vi "Periodic 1-Exp Distributed Random Variable.vi"(6 "seed":i32=-1, 8 "Error In":errorcluster, 9 "T":dbl, 10 "tau":dbl, 11 "# Elements":i32) -> (0 "Error Out":errorcluster, 3 "t Array":dbl[](array[numeric]))   [LabVIEW 2021, in "Math.lvlib"]
uses:
  Math.lvlib
  <vilib>/Utility/error.llb/Error Cluster From Error Code.vi
  <vilib>/gmath/statdist.llb/Uniform Random.vi
  <vilib>/ErrorRing/Error Ring.xnode
  <vilib>/gmath/NI_Gmath.lvlib
  Error/Error.lvlib
  Comparison/Comparison.lvlib
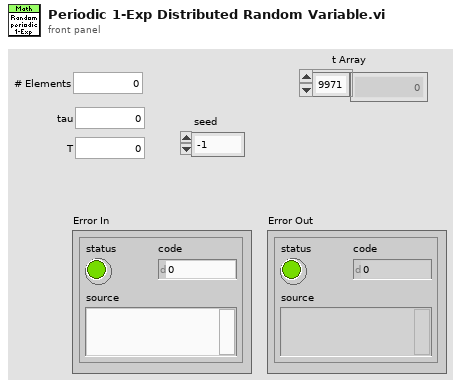
[diagram p1: front panel]
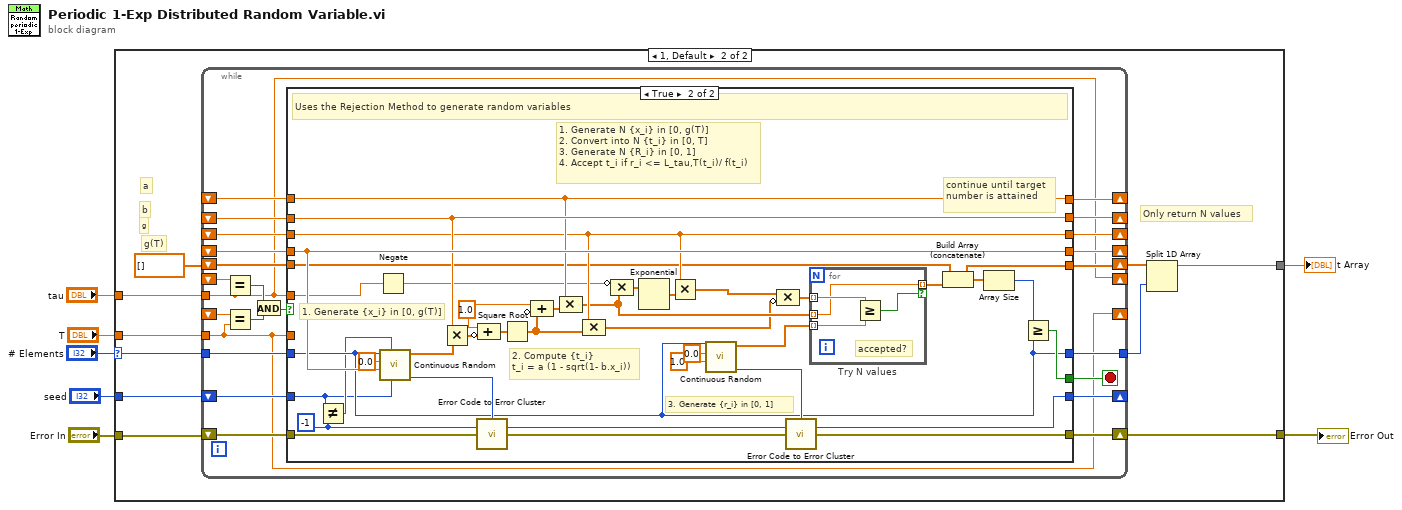
[diagram p0: block diagram]
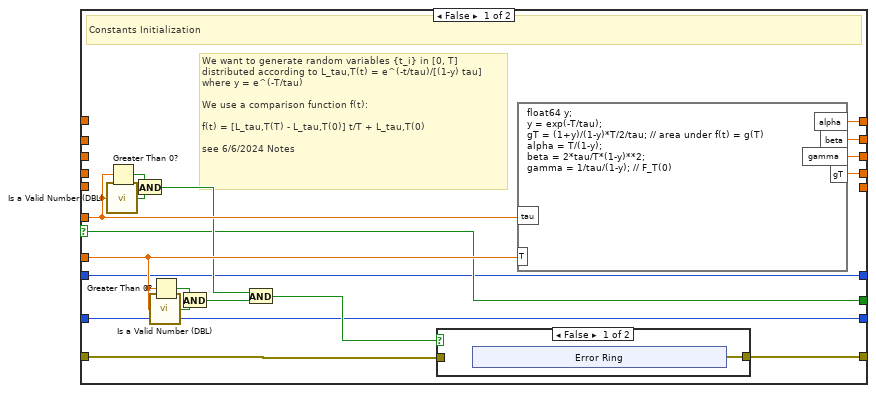
[diagram p3: hidden frame]
diagram:
  n1 = case shown="1, Default" "# Elements" {
    selector: "# Elements" -> [_ w16]
    tunnel: "tau" -> [_ w18]
    tunnel: "T" -> [_ w17]
    tunnel: "seed" -> [_ w15]
    tunnel: "Error In" -> [w8 w14]
    tunnel: [w8 w13] -> w2
    tunnel: [_ w10] -> w1
    frame 0 {
    }
    frame 1, Default {
      # "Only return N values"
      # "a"
      # "g"
      # "b"
      # "g(T)"
      n2 = while {
        tunnel: w18 -> [w19]
        shift-right: [w19] -> _
        shift-left: _ -> [w42]
        tunnel: w17 -> [w20]
        shift-right: [w20] -> _
        shift-left: _ -> [w41]
        shift-right: [w37] -> _
        shift-left: _ -> [w36]
        tunnel: w16 -> [w35]
        shift-right: [w34] -> _
        shift-left: _ -> [w32]
        shift-right: [w33] -> _
        shift-left: _ -> [w31]
        shift-right: [w28] -> w13
        shift-left: w14 -> [w29]
        shift-right: [w27] -> _
        shift-left: _ -> [w26]
        shift-right: [w23] -> w12
        shift-left: dbl[] [] -> [w24]
        tunnel: [w22] -> w11
        shift-right: [w21] -> _
        shift-left: w15 -> [w30]
        stop <- w25 stop-if-true
        n3 = Equal?(x=w42, y=w19) -> (x = y?=w39:bool)
        n4 = Equal?(x=w41, y=w20) -> (x = y?=w40:bool)
        n5 = And(x=w39, y=w40) -> (x .and. y?=w38:bool)
        n6 = case shown="True" w38 {
          selector: w38 -> [w45 _]
          tunnel: w19 -> [w57 w89]
          tunnel: w20 -> [w56 _]
          tunnel: [w60 w101] -> w37
          tunnel: w36 -> [_ w101]
          tunnel: w35 -> [w44 w73]
          tunnel: [w59 w99] -> w34
          tunnel: [w58 w90] -> w33
          tunnel: w32 -> [_ w99]
          tunnel: w31 -> [_ w90]
          tunnel: w30 -> [w43 w71]
          tunnel: w29 -> [w48 w69]
          tunnel: [w47 w67] -> w28
          tunnel: [w46 w92] -> w27
          tunnel: w26 -> [_ w92]
          tunnel: [w45 w84] -> w25
          tunnel: w24 -> [_ w86]
          tunnel: [_ w83] -> w23
          tunnel: [w44 w73] -> w22
          tunnel: [w43 w70] -> w21
          frame False {
            # "We want to generate random variables {t_i} in [0, T]\ndistributed according to L_tau,T(t) = e^(-t/tau)/[(1-y) tau]\nwhere y = e^(-T/tau)\n\nWe use a comparison function f(t):\n\nf(t) = [L_tau,T(T) - L_tau,T(0)] t/T + L_tau,T(0)\n\nsee 6/6/2024 Notes"
            # "Constants Initialization"
            n7 = call "Is a Valid Number (DBL).vi"("Number"=w57) -> ("Valid Number?"=w54:bool)  [unwired: 8 in]
            n8 = Greater Than 0?(x=w57) -> (x > 0?=w55:bool)
            n9 = And(x=w55, y=w54) -> (x .and. y?=w50:bool)
            n10 = call "Is a Valid Number (DBL).vi"("Number"=w56) -> ("Valid Number?"=w52:bool)  [unwired: 8 in]
            n11 = Greater Than 0?(x=w56) -> (x > 0?=w53:bool)
            n12 = And(x=w53, y=w52) -> (x .and. y?=w51:bool)
            n13 = And(x=w50, y=w51) -> (x .and. y?=w49:bool)
            n14 = case shown="False" w49 {
              tunnel: w48 -> [_ w66]
              tunnel: [w61 w66] -> w47
              frame False {
                n15 = xnode "Error Ring"() -> ("error out"=w61:errorcluster)
              }
              frame True {
              }
            }
            n16 = formula code="float64 y;\ny = exp(-T/tau);\ngT = (1+y)/(1-y)*T/2/tau; // area under f(t) = g(T)\nalpha = T/(1-y);\nbeta = 2*tau/T*(1-y)**2;\ngamma = 1/tau/(1-y); // F_T(0)"("tau"=w57, "T"=w56) -> ("gT"=w60:dbl, "beta"=w59:dbl, "gamma"=w58:dbl, "alpha"=w46:dbl)
          }
          frame True {
            w70 = -1 ("x")
            w94 = 1.0 ("xmin")
            # "3. Generate {r_i} in [0, 1]"
            # "2. Compute {t_i}\nt_i = a (1 - sqrt(1- b.x_i))"
            # "1. Generate {x_i} in [0, g(T)]"
            # "1. Generate N {x_i} in [0, g(T)]\n2. Convert into N {t_i} in [0, T]\n3. Generate N {R_i} in [0, 1]\n4. Accept t_i if r_i <= L_tau,T(t_i)/ f(t_i)"
            # "continue until target number is attained"
            # "Uses the Rejection Method to generate random variables"
            n17 = Not Equal?(x=w71, y=w70) -> (x != y?=w72:bool)
            n18 = Negate(x=w89) -> (-x=w81:dbl)
            n19 = call-poly <vilib>:"Continuous Random.vi"("seed"=w71, "reset"=w72, "xmax"=w101, "xmin"=0.0, "samples"=w73) -> ("error"=w96:i32, "uniform random data"=w100:dbl[])  [unwired: 5 in]
            n20 = Multiply(x=w99, y=w100) -> (x*y=w98:dbl[])
            n21 = call "Error Code to Error Cluster.vi"("Error Code"=w96, "Error In"=w69) -> ("Error Out"=w68:errorcluster)  [unwired: 13 in]
            n22 = Compound Arithmetic op=ADD(w94, invert w98) -> (w97:dbl[])
            n23 = Square Root(x=w97) -> (sqrt(x)=w95:dbl[])
            n24 = Compound Arithmetic op=ADD(w94, invert w95) -> (w93:dbl[])
            n25 = Compound Arithmetic op=MULTIPLY(w92, w93) -> (w80:dbl[])
            n26 = Compound Arithmetic op=MULTIPLY(w90, w95) -> (w78:dbl[])
            n27 = Compound Arithmetic op=MULTIPLY(invert w81, w80) -> (w82:dbl[])
            n28 = Exponential(1:w82) -> (0:w91:dbl[])
            n29 = Multiply(x=w90, y=w91) -> (x*y=w88:dbl[])
            n30 = call-poly <vilib>:"Continuous Random.vi"("xmax"=1.0, "xmin"=0.0 ("xmax"), "samples"=w73) -> ("error"=w75:i32, "uniform random data"=w76:dbl[])  [unwired: 7 in]
            n31 = Compound Arithmetic op=MULTIPLY(w88, invert w78) -> (w79:dbl[])
            n32 = call "Error Code to Error Cluster.vi"("Error Code"=w75, "Error In"=w68) -> ("Error Out"=w67:errorcluster)  [unwired: 13 in]
            n33 = for "Try N values" {
              tunnel: [w105] -> w87 mode=indexing if=w103
              tunnel: w79 -> [w106] mode=indexing
              tunnel: w80 -> [w105] mode=indexing
              tunnel: w76 -> [w104] mode=indexing
              # "accepted?"
              n34 = Greater Or Equal?(x=w106, y=w104) -> (x >= y?=w103:bool)
            }
            n35 = Build Array (concatenate)(w86, w87) -> (w83:dbl[])
            n36 = Array Size(array=w83) -> (size(s)=w85:i32)
            n37 = Greater Or Equal?(x=w85, y=w73) -> (x >= y?=w84:bool)
          }
        }
      }
      n38 = Split 1D Array(array=w12, index=w11) -> (first subarray=w10:dbl[])  [unwired: 1 out]
    }
  }
  "t Array" <- w1
  "Error Out" <- w2
